vi "2015 Network Variables.vi"(9 "ERD_Always Show":T3, 10 "Board Index Startup":i32, 11 "Serial Number":string) -> ()   [LabVIEW 2014]
uses:
  Washer Soft Load Box/type defs/ERD_Always_Show.ctl
  Washer Soft Load Box/type defs/Redundant.ctl
  Washer Soft Load Box/type defs/Version.ctl
panel:
  in  "Version":T1
  in  "Redundant Micro":T2
  # "Software Version"
  # "Critical Version"
  # "Non-Critical"
  # "XML Crit Ver"
  # "XML Non-Crit"
  # "Daily Build"
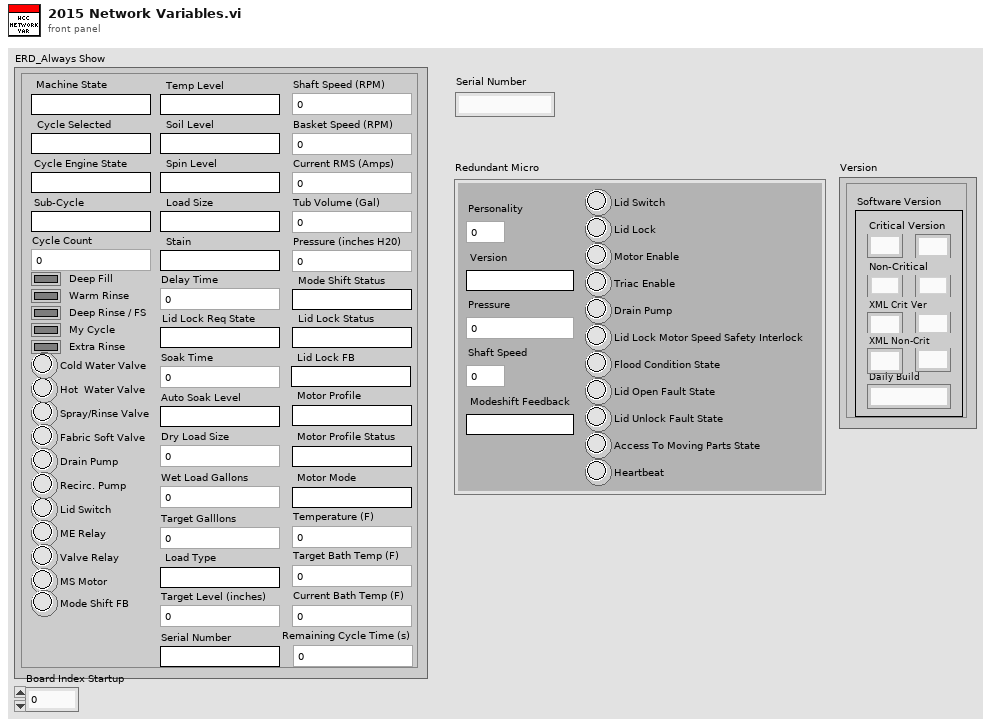
[diagram p1: front panel]
types:
  T1 = typedef "Version.ctl" = cluster{"Critical Major":string, "Critical Minor":string, "Non-Critical Minor":string, "Non-Critical Major":string, "XML Crit Minor":string, "XMLCrit Major":string, "Daily Rev":string, "XML Non-crit Minor":string, "Xml Non-crit Major":string}
  T2 = typedef "Redundant.ctl" = cluster{"Version":string, "Personality":u8, "Pressure ":dbl, "Shaft Speed":u16, "Modeshift Feedback":string, "Lid Switch":bool, "Lid Lock":bool, "Triac Enable":bool, "Drain Pump":bool, "Lid Lock Motor Speed Safety Interlock":bool, "Flood Condition State":bool, "Lid Open Fault State":bool, "Access To Moving Parts State":bool, "Heartbeat":bool, "Motor Enable":bool, "Lid Unlock Fault State":bool}
  T3 = typedef "ERD_Always_Show.ctl" = cluster{"Basket Speed (RPM)":u16, "Machine State":string, "Tub Volume (Gal)":dbl, "Pressure (inches H20)":dbl, "Lid Switch ":bool, "Current RMS (Amps)":dbl, "Cycle Selected":string, "Lid Lock Status":string, "Mode Shift Status":string, "Spray/Rinse Valve":bool, "Fabric Soft Valve":bool, "Drain Pump":bool, "Recirc. Pump":bool, "Cycle Engine State":string, "Hot  Water Valve":bool, "Cold Water Valve":bool, "Motor Profile":string, "Motor Profile Status":string, "Motor Mode":string, "ME Relay":bool, "Cycle Count":u32, "Deep Rinse / FS":bool, "My Cycle":bool, "Soil Level":string, "Spin Level":string, "Stain":string, "Temp Level":string, "Load Size":string, "Delay Time":u16, "Soak Time":u16, "Deep Fill":bool, "Warm Rinse":bool, "Auto Soak Level":string, "Extra Rinse":bool, "Wet Load Gallons":dbl, "Target Galllons":dbl, "Sub-Cycle":string, "Load Type":string, "Target Level (inches)":u32, "Valve Relay":bool, "Dry Load Size":dbl, "Shaft Speed (RPM) ":u16, "MS Motor":bool, "Mode Shift FB":bool, "Target Bath Temp (F)":dbl, "Temperature (F)":dbl, "Current Bath Temp (F)":dbl, "Lid Lock FB":string, "Lid Lock Req State":string, "Remaining Cycle Time (s)":dbl, "Serial Number":string}
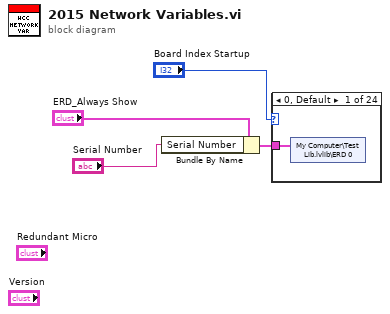
[diagram p0: block diagram]
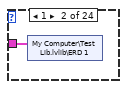
[diagram p2: hidden frame]
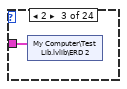
[diagram p3: hidden frame]
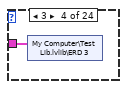
[diagram p4: hidden frame]
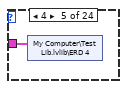
[diagram p5: hidden frame]
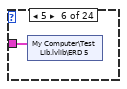
[diagram p6: hidden frame]
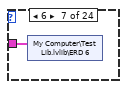
[diagram p7: hidden frame]
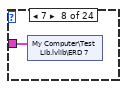
[diagram p8: hidden frame]
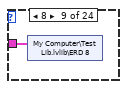
[diagram p9: hidden frame]
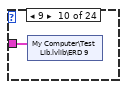
[diagram p10: hidden frame]
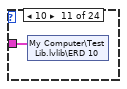
[diagram p11: hidden frame]
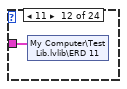
[diagram p12: hidden frame]
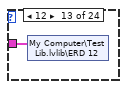
[diagram p13: hidden frame]
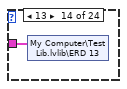
[diagram p14: hidden frame]
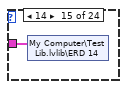
[diagram p15: hidden frame]
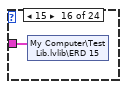
[diagram p16: hidden frame]
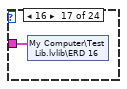
[diagram p17: hidden frame]
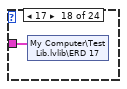
[diagram p18: hidden frame]
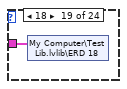
[diagram p19: hidden frame]
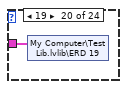
[diagram p20: hidden frame]
diagram:
  n1 = Bundle By Name(cluster="ERD_Always Show", "Serial Number"="Serial Number") -> (w1:T3)
  n2 = case shown="0, Default" "Board Index Startup" {
    tunnel: w1 -> [w5 w6 w7 w8 w9 w10 w11 w12 w13 w14 w15 w16 w17 w18 w19 w20 w21 w22 w23 w24 w25 w26 w27 w28]
    frame 0, Default {
      n3 = shared-variable "My Computer\\Test Lib.lvlib\\ERD 0"(w5) -> ()  [unwired: 1 in, 1 out]
    }
    frame 1 {
      n4 = shared-variable "My Computer\\Test Lib.lvlib\\ERD 1"(w6) -> ()  [unwired: 1 in, 1 out]
    }
    frame 2 {
      n5 = shared-variable "My Computer\\Test Lib.lvlib\\ERD 2"(w7) -> ()  [unwired: 1 in, 1 out]
    }
    frame 3 {
      n6 = shared-variable "My Computer\\Test Lib.lvlib\\ERD 3"(w8) -> ()  [unwired: 1 in, 1 out]
    }
    frame 4 {
      n7 = shared-variable "My Computer\\Test Lib.lvlib\\ERD 4"(w9) -> ()  [unwired: 1 in, 1 out]
    }
    frame 5 {
      n8 = shared-variable "My Computer\\Test Lib.lvlib\\ERD 5"(w10) -> ()  [unwired: 1 in, 1 out]
    }
    frame 6 {
      n9 = shared-variable "My Computer\\Test Lib.lvlib\\ERD 6"(w11) -> ()  [unwired: 1 in, 1 out]
    }
    frame 7 {
      n10 = shared-variable "My Computer\\Test Lib.lvlib\\ERD 7"(w12) -> ()  [unwired: 1 in, 1 out]
    }
    frame 8 {
      n11 = shared-variable "My Computer\\Test Lib.lvlib\\ERD 8"(w13) -> ()  [unwired: 1 in, 1 out]
    }
    frame 9 {
      n12 = shared-variable "My Computer\\Test Lib.lvlib\\ERD 9"(w14) -> ()  [unwired: 1 in, 1 out]
    }
    frame 10 {
      n13 = shared-variable "My Computer\\Test Lib.lvlib\\ERD 10"(w15) -> ()  [unwired: 1 in, 1 out]
    }
    frame 11 {
      n14 = shared-variable "My Computer\\Test Lib.lvlib\\ERD 11"(w16) -> ()  [unwired: 1 in, 1 out]
    }
    frame 12 {
      n15 = shared-variable "My Computer\\Test Lib.lvlib\\ERD 12"(w17) -> ()  [unwired: 1 in, 1 out]
    }
    frame 13 {
      n16 = shared-variable "My Computer\\Test Lib.lvlib\\ERD 13"(w18) -> ()  [unwired: 1 in, 1 out]
    }
    frame 14 {
      n17 = shared-variable "My Computer\\Test Lib.lvlib\\ERD 14"(w19) -> ()  [unwired: 1 in, 1 out]
    }
    frame 15 {
      n18 = shared-variable "My Computer\\Test Lib.lvlib\\ERD 15"(w20) -> ()  [unwired: 1 in, 1 out]
    }
    frame 16 {
      n19 = shared-variable "My Computer\\Test Lib.lvlib\\ERD 16"(w21) -> ()  [unwired: 1 in, 1 out]
    }
    frame 17 {
      n20 = shared-variable "My Computer\\Test Lib.lvlib\\ERD 17"(w22) -> ()  [unwired: 1 in, 1 out]
    }
    frame 18 {
      n21 = shared-variable "My Computer\\Test Lib.lvlib\\ERD 18"(w23) -> ()  [unwired: 1 in, 1 out]
    }
    frame 19 {
      n22 = shared-variable "My Computer\\Test Lib.lvlib\\ERD 19"(w24) -> ()  [unwired: 1 in, 1 out]
    }
    frame 20 {
      n23 = shared-variable "My Computer\\Test Lib.lvlib\\ERD 20"(w25) -> ()  [unwired: 1 in, 1 out]
    }
    frame 21 {
      n24 = shared-variable "My Computer\\Test Lib.lvlib\\ERD 21"(w26) -> ()  [unwired: 1 in, 1 out]
    }
    frame 22 {
      n25 = shared-variable "My Computer\\Test Lib.lvlib\\ERD 22"(w27) -> ()  [unwired: 1 in, 1 out]
    }
    frame 23 {
      n26 = shared-variable "My Computer\\Test Lib.lvlib\\ERD 23"(w28) -> ()  [unwired: 1 in, 1 out]
    }
  }
